vi "sub vi - send mail with attach v2.vi"(5 "subject":string, 6 "Attachements":path[](array[path]), 7 "send address":string) -> (0 "error out":errorcluster)   [LabVIEW 2013]
uses:
  <vilib>/smtpClient/Set Message Text.vi
  <vilib>/smtpClient/LabVIEWSMTPClient.lvlib
panel:
  in  "Array - send address string":string[](array[string])
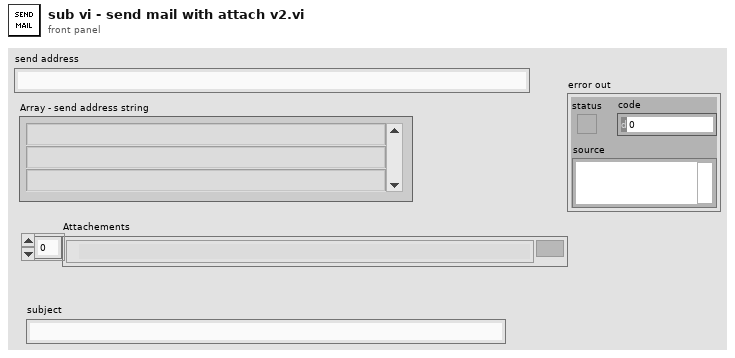
[diagram p1: front panel]
types:
  T1 = typedef "LabVIEWSMTPClient.lvlib/SmtpClientHandle.ctl" = refnum<k1>
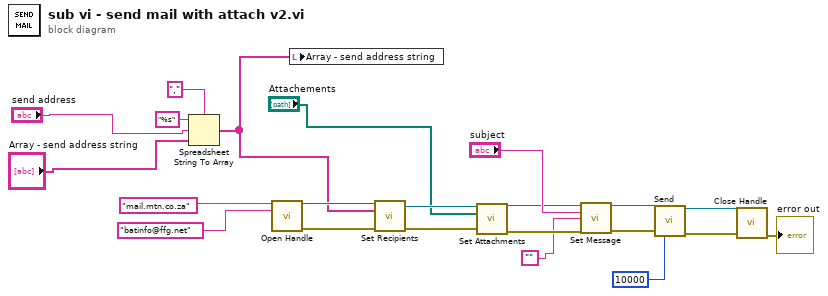
[diagram p0: block diagram]
diagram:
  n1 = Spreadsheet String To Array(delimiter (Tab)=",", format string="%s", spreadsheet string="send address", array type (2D Dbl)="Array - send address string") -> (array=w2:string[])
  n2 = call <vilib>:"Open Handle.vi"("server address"="mail.mtn.co.za", "from"="batinfo@ffg.net") -> ("handle out"=w20:T1, "error out"=w19:errorcluster)  [unwired: 12 in]
  n3 = local write "Array - send address string"(w2) -> ()
  n4 = call <vilib>:"Set Recipients.vi"("handle in"=w20, "to"=w2, "error in (no error)"=w19) -> ("handle out"=w18:T1, "error out"=w14:errorcluster)  [unwired: 11 in]
  n5 = call <vilib>:"Set Attachments.vi"("handle in"=w18, "attachments"="Attachements", "error in (no error)"=w14) -> ("handle out"=w16:T1, "error out"=w13:errorcluster)  [unwired: 11 in]
  n6 = call-poly <vilib>:"Set Message.vi"("handle in"=w16, "subject"="subject", "plain text message"="", "error in (no error)"=w13) -> ("handle out"=w15:T1, "error out"=w12:errorcluster)  [unwired: 10 in]
  n7 = call <vilib>:"Send.vi"("handle in"=w15, "error in (no error)"=w12, "timeout in ms (10000)"=10000) -> ("handle out"=w11:T1, "error out"=w10:errorcluster)  [unwired: 10 in, 1 out]
  n8 = call <vilib>:"Close Handle.vi"("handle in"=w11, "error in (no error)"=w10) -> ("error out"=→"error out":errorcluster)  [unwired: 12 in, 1 out]
